vi "queStartup.vi"(0 "object in":refnum<class "interface.lvclass">, 1 "启动文件路径":path, 5 "error in (no error)":errorcluster) -> (14 "object out":refnum<class "interface.lvclass">, 15 "包含启动项":bool, 16 "启动文件路径":path, 19 "error out":errorcluster)   [LabVIEW 2016, in "interface.lvclass"]
uses:
  interface.lvclass
  <vilib>/registry/registry.llb/Registry RtKey.ctl
  <vilib>/registry/registry.llb/Read Registry Value Simple STR.vi
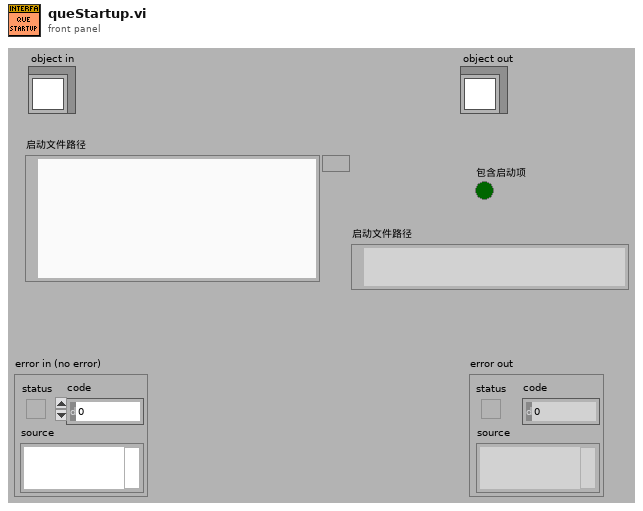
[diagram p1: front panel]
types:
  T1 = typedef "Registry RtKey.ctl" = enum32{"HKEY_CLASSES_ROOT", "HKEY_CURRENT_USER", "HKEY_LOCAL_MACHINE", "HKEY_USERS", "HKEY_PERFORMANCE_DATA", "HKEY_CURRENT_CONFIG", "HKEY_DYN_DATA"}
  T2 = typedef "Registry refnum.ctl" = refnum<k1>
  T3 = cluster{"numValues":i32, "maxValueNameLen":i32, "maxValueDataLen":i32}
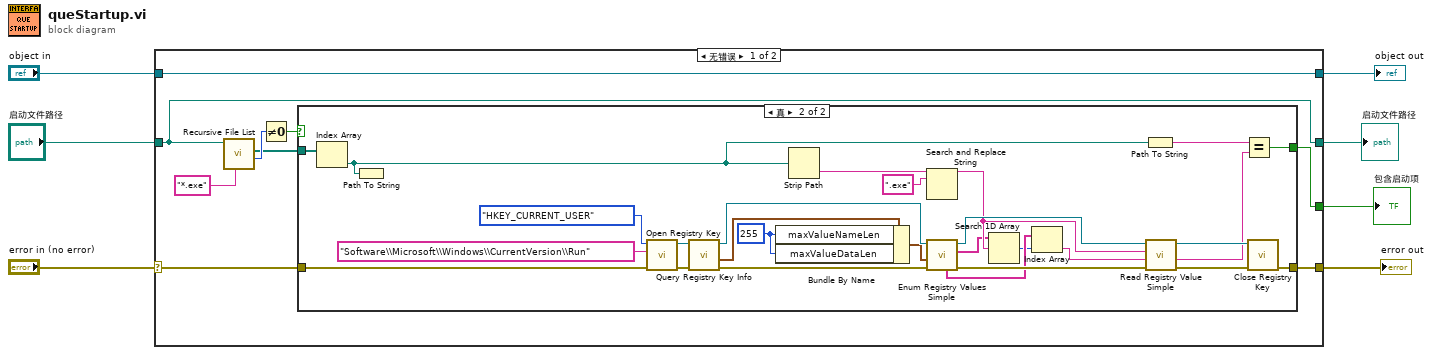
[diagram p0: block diagram]
diagram:
  n1 = case shown="无错误" "error in (no error)" {
    selector: "error in (no error)" -> [w11 w47]
    tunnel: [w10 w47] -> w6
    tunnel: [w16 w46] -> w4
    tunnel: "object in" -> [w16 w46]
    tunnel: "启动文件路径" -> [w8 w45]
    tunnel: [w9 _] -> w2
    tunnel: [w8 w45] -> w1
    frame No Error {
      n2 = call <vilib>:"Recursive File List.vi"("pattern"="*.exe", "Folder Path"=w8) -> ("Number of Files"=w14:i32, "All Files in Dir"=w13:path[])  [unwired: 5 in, 3 out]
      n3 = Not Equal To 0?(x=w14) -> (x != 0?=w15:bool)
      n4 = case shown="真" w15 {
        tunnel: w13 -> [_ w44]
        tunnel: [_ w26] -> w9
        tunnel: w11 -> [w17 w19]
        tunnel: [w17 w18] -> w10
        frame False {
        }
        frame True {
          w20 = 255 ("maxValueNameLen")
          n5 = Index Array(array=w44) -> (element=w25:path)  [unwired: 1 in]
          n6 = Path To String(path=w25) -> ()  [unwired: 1 out]
          n7 = call <vilib>:"Open Registry Key.vi"("error in (no error)"=w19, "subkey"="Software\\Microsoft\\Windows\\CurrentVersion\\Run", "root key (HKEY_LOCAL_MACHINE)"=Registry_RtKey."HKEY_CURRENT_USER") -> ("error out"=w38:errorcluster, "refnum out"=w39:T2)  [unwired: 7 in]
          n8 = call <vilib>:"Query Registry Key Info.vi"("error in (no error)"=w38, "refnum"=w39) -> ("error out"=w36:errorcluster, "value info"=w22:T3, "refnum out"=w37:T2)  [unwired: 5 in, 2 out]
          n9 = Bundle By Name(cluster=w22, "maxValueNameLen"=w20, "maxValueDataLen"=w20) -> (w21:T3)
          n10 = Strip Path(path=w25) -> (name=w43:string)  [unwired: 1 out]
          n11 = Search and Replace String(input string=w43, search string=".exe" ("搜索字符串")) -> (result string=w31:string)  [unwired: 6 in, 3 out]
          n12 = call <vilib>:"Enum Registry Values Simple.vi"("error in (no error)"=w36, "value info"=w21, "refnum"=w37) -> ("error out"=w33:errorcluster, "values"=w30:string[], "refnum out"=w35:T2, "String/Binary data"=w29:string[])  [unwired: 3 in, 2 out]
          n13 = Search 1D Array(1D array=w30, element=w31) -> (index of element=w27:i32)  [unwired: 1 in]
          n14 = Index Array(array=w29, index=w27) -> (element=w28:string)
          n15 = Path To String(path=w25) -> (string=w24:string)
          n16 = call-poly <vilib>:"Read Registry Value Simple.vi"("error in (no error)"=w33, "default data"=w28, "value"=w31, "refnum"=w35) -> ("error out"=w32:errorcluster, "String/Binary data"=w23:string, "refnum out"=w34:T2)  [unwired: 2 in, 1 out]
          n17 = Equal?(x=w24, y=w23) -> (x = y?=w26:bool)
          n18 = call <vilib>:"Close Registry Key.vi"("error in (no error)"=w32, "refnum"=w34) -> ("error out"=w18:errorcluster)  [unwired: 5 in]
        }
      }
    }
    frame Error {
    }
  }
  "error out" <- w6
  "object out" <- w4
  "包含启动项" <- w2
  "启动文件路径" <- w1
